vi "SetRenderTarget.vi"(8 "No Error":errorcluster, 10 "Texture [SDL_Texture *]":T1 format="%.0x", 11 "Renderer [SDL_Renderer *]":T2 format="%.0x") -> (0 "error out":errorcluster)   [LabVIEW 2026, in "SDL3.lvlib" / "Render.lvlib"]
doc: "<B>Summary</B>\nSet a texture as the current rendering target.\n\n<B>Remarks</B>\nThe default render target is the window for which the renderer was created. To stop rendering to a texture and render to the window again, call this function with a NULL texture."
uses:
  Render.lvlib
  <vilib>/Utility/error.llb/Error Cluster From Error Code.vi
  Error/Error.lvlib
  Lib/SDL3.dll
  SDL_Renderer--pointer.ctl
  SDL_Texture--pointer.ctl
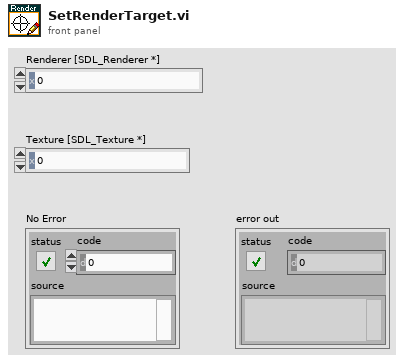
[diagram p1: front panel]
types:
  T1 = typedef "SDL3.lvlib/Render.lvlib/SDL_Texture--pointer.ctl" = i64
  T2 = typedef "SDL3.lvlib/Render.lvlib/SDL_Renderer--pointer.ctl" = i64
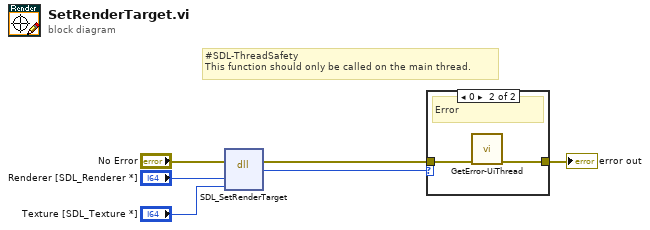
[diagram p0: block diagram]
diagram:
  # "#SDL-ThreadSafety\nThis function should only be called on the main thread."
  n1 = dll-call lib="C:/Users/saukko/Dev/LV-SDL3/Sources/SDL3/Lib/SDL3.*" fn="SDL_SetRenderTarget"(error in="No Error", "renderer"="Renderer [SDL_Renderer *]", "texture"="Texture [SDL_Texture *]") -> (error out=w2:errorcluster, "return type"=w1:i32)  [unwired: 4 in, 1 out]
  n2 = case shown="0" w1 {
    tunnel: w2 -> [w7 w9]
    tunnel: [w7 w8] -> w5
    frame Default {
      # "Ok"
    }
    frame 0 {
      # "Error"
      n3 = call "GetError-UiThread.vi"("No Error"=w9) -> ("error out"=w8:errorcluster)  [unwired: 10 in]
    }
  }
  "error out" <- w5
